vi "Untitled 2.vi"() -> ()   [LabVIEW 2018]
panel:
  in  "Table Control":string[][](table)
  out "Array 3":i32[](array[numeric])
  out "Array":i32[](array[numeric])
  out "Array 2":i32[](array[numeric])
  out "error out":errorcluster
  in  "error in (no error)":errorcluster
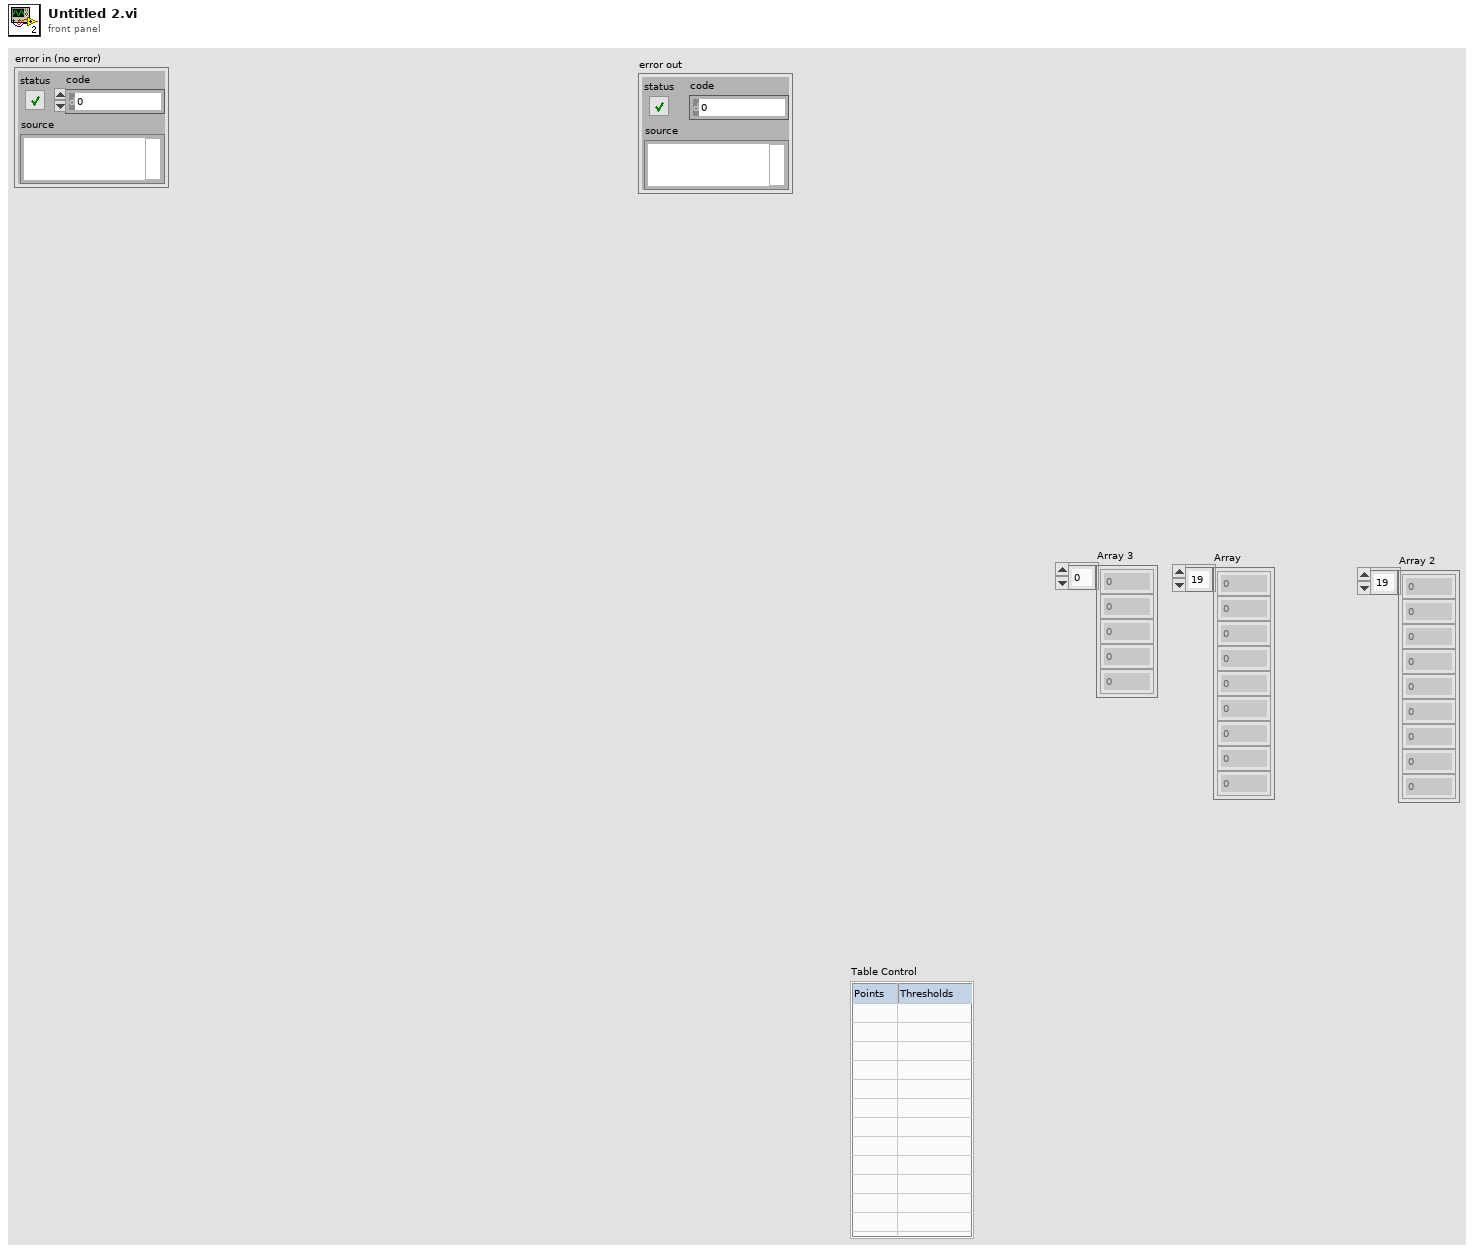
[diagram p1: front panel]
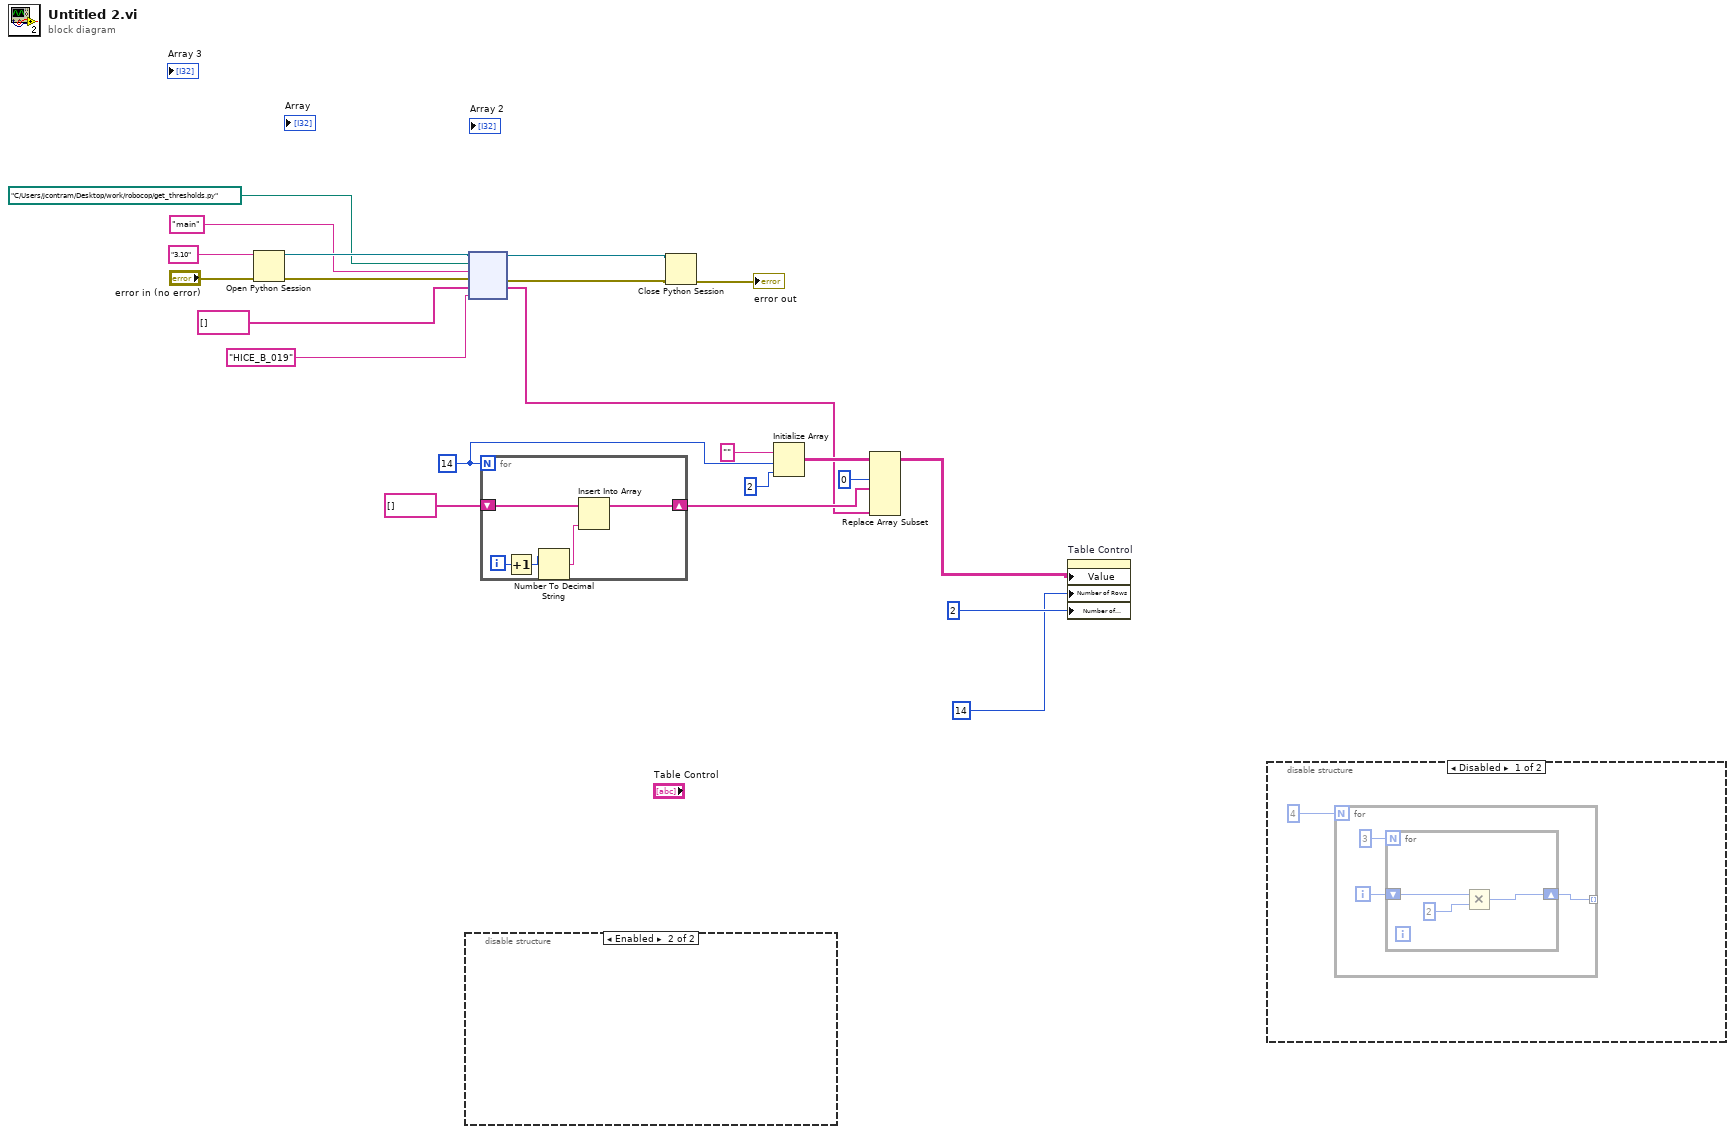
[diagram p0: block diagram]
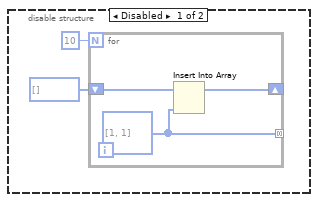
[diagram p2: hidden frame]
diagram:
  w6 = 14 ("dimension size")
  n1 = Open Python Session(python version="3.10" ("Python version"), 3:"error in (no error)") -> (session out=w22:refnum<k35>, error out=w20:errorcluster)  [unwired: 1 in]
  n2 = disable-structure shown="Enabled" {
    frame Disabled {
      n3 = for {
        N: 10 -> [_]
        shift-right: [w28] -> w24
        shift-left: i32[] [] -> [w29]
        tunnel: [w27] -> w23 mode=concatenating
        w27 = i32[] [1, 1]
        n4 = Insert Into Array(array=w29, new element=w27) -> (w28:i32[])  [unwired: 1 in]
      }
    }
    frame Enabled {
    }
  }
  n5 = node(w22, path "C:/Users/jcontram/Desktop/work/robocop/get_thresholds.py" ("module path"), "main" ("function name"), w20, string[] [], "HICE_B_019") -> (w21:refnum<k35>, w19:errorcluster, w5:string[])  [unwired: 1 in, 2 out]
  n6 = for {
    N: w6 -> [_]
    shift-right: [w33] -> w7
    shift-left: string[] [] -> [w34]
    i -> [w32]
    n7 = Increment(x=w32) -> (x+1=w30:i32)
    n8 = Number To Decimal String(number=w30) -> (decimal integer string=w31:string)  [unwired: 1 in]
    n9 = Insert Into Array(array=w34, new element=w31) -> (w33:string[])  [unwired: 1 in]
  }
  n10 = Close Python Session(session in=w21, error in=w19) -> (11:→"error out":errorcluster)
  n11 = Initialize Array("", w6, 2 ("dimension size")) -> (w9:string[][])
  n12 = Replace Array Subset(array=w9, new element #1=w7, index (col) #1=0 ("disabled index (col)"), new element #2=w5) -> (w1:string[][])  [unwired: 3 in]
  n13 = property on="Table Control" class="Tbl (strict)"("Value"=w1, "Number of Rows"=14, "Number of Columns"=2) -> ()  [unwired: 2 in, 2 out]
  n14 = disable-structure shown="Disabled" {
    frame Disabled {
      n15 = for {
        N: 4 -> [_]
        tunnel: [w37] -> w35 mode=indexing
        i -> [w38]
        n16 = for {
          N: 3 -> [_]
          shift-right: [w40] -> w37
          shift-left: w38 -> [w41]
          n17 = Multiply(x=w41, y=2) -> (x*y=w40:i32)
        }
      }
    }
    frame Enabled {
    }
  }
